vi "Init.vi"(8 "error in (no error)":errorcluster) -> (0 "error out":errorcluster)   [LabVIEW 2017]
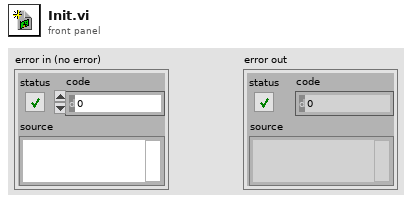
[diagram p1: front panel]
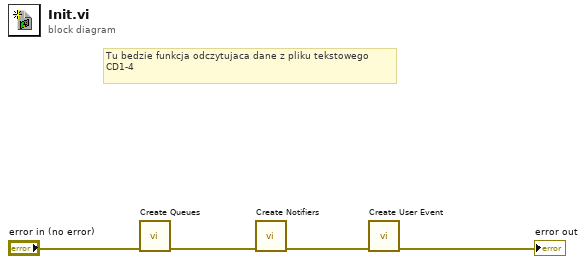
[diagram p0: block diagram]
diagram:
  # "Tu bedzie funkcja odczytujaca dane z pliku tekstowego\nCD1-4"
  n1 = call "Create Queues.vi"("Error In"="error in (no error)") -> ("Error Out"=w3:errorcluster)  [unwired: 10 in]
  n2 = call "Create Notifiers.vi"("error in (no error)"=w3) -> ("error out"=w2:errorcluster)  [unwired: 10 in]
  n3 = call "Create User Event.vi"("Error In"=w2) -> ("Error Out"=→"error out":errorcluster)  [unwired: 10 in]
